vi "getpassfromfile.vi"() -> (1 "line string":string)   [LabVIEW 2013]
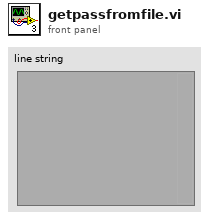
[diagram p1: front panel]
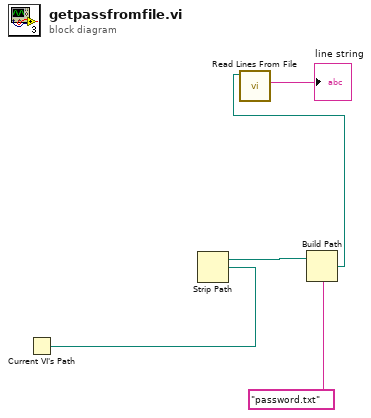
[diagram p0: block diagram]
diagram:
  n1 = Current VI's Path() -> (path=w2:path)
  n2 = Strip Path(path=w2) -> (stripped path=w3:path)  [unwired: 1 out]
  n3 = Build Path(base path=w3, name or relative path="password.txt") -> (appended path=w5:path)
  n4 = call <vilib>:"Read Lines From File.vi"("file path (dialog if empty)"=w5) -> ("line string"=→"line string":string)  [unwired: 5 in, 3 out]
